vi "AndorAcqSingleImgToTiffStack.vi"(6 "Image Nr":i32, 7 "Total Images":i32, 8 "error in (no error)":errorcluster, 9 "Exposure":sgl=50.0 format="%#_g ms", 10 "Image Name":string, 11 "TiffHandle IN":refnum<k24>) -> (0 "error out":errorcluster, 2 "Image":T1, 3 "TiffOut":refnum<k24>)   [LabVIEW 2018, in "AndorOWN.lvlib"]
uses:
  AndorOWN.lvlib
  C:/Users/e14user/Documents/LabVIEW software/GitRepo/lib/tiff/LVTiffWriter/BitMiracle.LibTiff.NET.dll
  tiff/LVTiffWriter/BitMiracle.LibTiff.NET.dll
  <vilib>/vision/Image Controls.llb/IMAQ Image.ctl
  Andor SDK/AndorSDK.lvlib
  tiff/LVTiffWriter/LVTiffWriter.lvlib
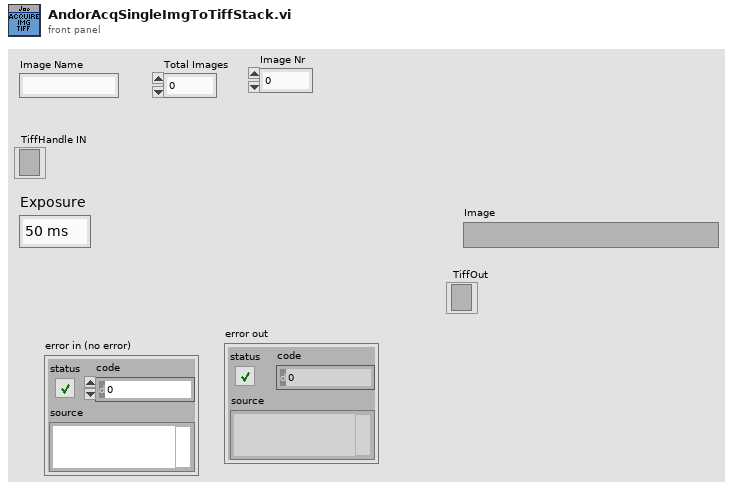
[diagram p1: front panel]
types:
  T1 = typedef "IMAQ Image.ctl" = refnum<image>
  T2 = typedef "Image Type" = u32
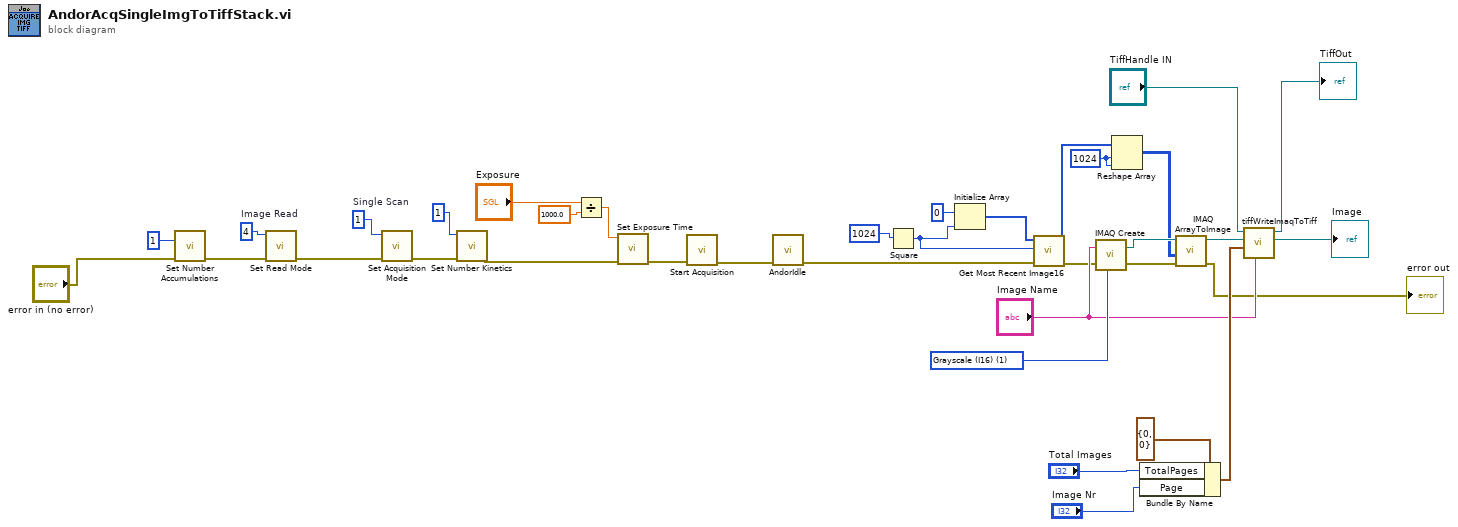
[diagram p0: block diagram]
diagram:
  w23 = T2 1 items=["Grayscale (U8)", "Grayscale (I16)", "Grayscale (SGL)", "Complex (CSG)", "RGB (U32)", "HSL (U32)", "RGB (U64)", "Grayscale (U16)"] ("Image Type")
  w22 = 1024 ("dimension size")
  w32 = 1  # Single Scan
  w35 = 4  # Image Read
  n1 = call "Set Number Accumulations.vi"("error in (no error)"="error in (no error)", "number"=1) -> ("error out"=w10:errorcluster)  [unwired: 8 in, 1 out]
  n2 = call "Set Read Mode.vi"("error in (no error)"=w10, "mode"=w35) -> ("error out"=w11:errorcluster)  [unwired: 8 in, 1 out]
  n3 = call "Set Acquisition Mode.vi"("error in (no error)"=w11, "mode"=w32) -> ("error out"=w9:errorcluster)  [unwired: 8 in, 1 out]
  n4 = call "Set Number Kinetics.vi"("error in (no error)"=w9, "number"=1) -> ("error out"=w8:errorcluster)  [unwired: 8 in, 1 out]
  n5 = Divide(x="Exposure", y=sgl 1000.0) -> (x/y=w30:sgl)
  n6 = call "Set Exposure Time.vi"("error in (no error)"=w8, "time"=w30) -> ("error out"=w7:errorcluster)  [unwired: 8 in, 1 out]
  n7 = call "Start Acquisition.vi"("error in (no error)"=w7) -> ("error out"=w6:errorcluster)  [unwired: 9 in, 1 out]
  n8 = call "AndorIdle.vi"("error in (no error)"=w6) -> ("error out"=w5:errorcluster)  [unwired: 9 in, 1 out]
  n9 = Square(x=u32 1024) -> (x^2=w25:u32)
  n10 = Initialize Array(i16 0 ("element"), w25) -> (w26:i16[])
  n11 = call "Get Most Recent Image16.vi"("error in (no error)"=w5, "size"=w25, "arr"=w26) -> ("error out"=w4:errorcluster, "arr out"=w36:i16[])  [unwired: 6 in, 1 out]
  n12 = call "IMAQ Create"("Image Name"="Image Name", "Image Type"=w23, "error in (no error)"=w4) -> ("New Image"=w24:T1, "error out"=w3:errorcluster)  [unwired: 2 in]
  n13 = Reshape Array(w36, w22, w22) -> (w12:i16[][])
  n14 = Bundle By Name(cluster=cluster{"Page":i32, "TotalPages":i32} {"Page"=0, "TotalPages"=0} ("Multipage"), "TotalPages"="Total Images", "Page"="Image Nr") -> (w16:cluster{"Page":i32, "TotalPages":i32})
  n15 = call "IMAQ ArrayToImage"("error in (no error)"=w3, "Image Pixels (I16)"=w12, "Image"=w24) -> ("error out"=→"error out":errorcluster, "Image Out"=w21:T1)  [unwired: 7 in]
  n16 = call "tiffWriteImaqToTiff.vi"("ImageDescription"="Image Name", "Multipage"=w16, "ImaqIn"=w21, "TiffIn"="TiffHandle IN") -> ("ImaqOut"=→"Image":T1, "TiffOut"=→"TiffOut":refnum<k24>)  [unwired: 6 in]
